vi "Constants.vi"() -> ()   [LabVIEW 2020, in "Routing and Faulting Shared.lvlib"]
doc: "Use this Global VI to access the GUIDs assigned to the page resources of the Custom Device."
uses:
  Dependencies.llb/Routing and Faulting Shared.lvlib
panel:
  in  "Tab Control":enum32{"GUIDS", "Constants", "Properties"}(tab)
  in  "Disabled Routing Channel GUID":string="d53b9e39-8c97-48d0-a889-a3e6598ed856"
  in  "Routing Channel GUID":string="7ecc8b72-3e89-41fd-aa1c-b993e8fe884f"
  in  "Status GUID":string="fafe2633-52e8-4be6-bb95-b07e42834d60"
  in  "Routing Channels GUID":string="ce8870b5-cb8e-4b52-ac34-5b792fdc2ead"
  in  "SLSC Switch GUID":string="5e47c8de-3ec6-490b-8897-5526d4aea756"
  in  "Endpoint Aliases GUID":string="58f3342d-82ee-4932-869a-6f49da3049e5"
  in  "Routing and Faulting GUID":string="4e591626-626d-4903-9a6e-1f2a7b879f4d"
  in  "Tip-Strip Update Period":dbl=0.1 format="%#_g s"
  in  "Duplicate Endpoint Message":string="Endpoint \"%s\" is already assigned to alias \"%s\"."
  in  "Duplicate Alias Message":string="Alias \"%s\" already exists for endpoint \"%s\"."
  in  "Routing Channel Default Name":string="Routing Channel"
  in  "Status Code":string="Status Code"
  in  "Heartbeat":string="Heartbeat"
  in  "Status":string="Status"
  in  "Hardware":string="Hardware"
  in  "Routing Channels":string="Routing Channels"
  in  "Endpoint Aliases":string="Endpoint Aliases"
  in  "Routing and Faulting Name":string="Routing and Faulting"
  in  "Previously Shown State":string="Previously Shown State"
  in  "Compiled.Settings":string="Compiled.Settings"
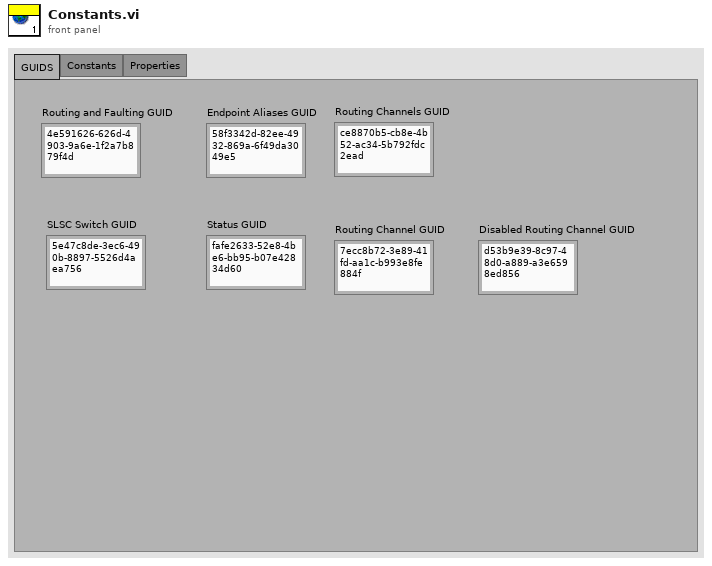
[diagram p1: front panel]
diagram:
